vi "Warn.vi"(8 "Error In":errorcluster, 11 "Text":string) -> (0 "Error Out":errorcluster)   [LabVIEW 2014, in "Logger.lvlib"]
uses:
  Logger.lvlib
  Private/_Logger Action.ctl
  Controls/Message.ctl
  Controls/Tag.ctl
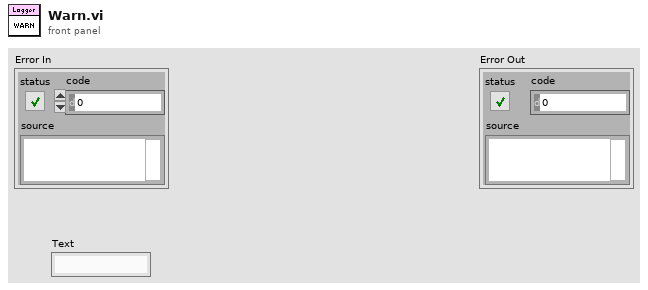
[diagram p1: front panel]
types:
  T1 = typedef "Logger.lvlib/Tag.ctl" = enum16{"Fatal", "Error", "Warn", "Info", "Debug", "Trace"}
  T2 = typedef "Logger.lvlib/_Logger Action.ctl" = enum16{"Initialize", "Register", "Log", "Unregister", "Set Level", "Shutdown"}
  T3 = typedef "Logger.lvlib/Message.ctl" = cluster{"Time Stamp":timestamp, "Tag":T1, "Source":string, "Text":string}
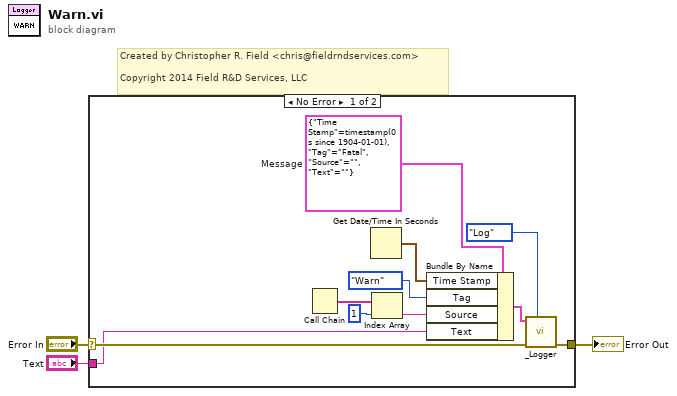
[diagram p0: block diagram]
diagram:
  # "Created by Christopher R. Field <chris@fieldrndservices.com>\n\nCopyright 2014 Field R&D Services, LLC"
  n1 = case shown="No Error" "Error In" {
    selector: "Error In" -> [w5 w15]
    tunnel: [w6 w15] -> w2
    tunnel: "Text" -> [w4 _]
    frame No Error {
      w11 = T3 {"Time Stamp"=timestamp(0 s since 1904-01-01), "Tag"=enum."Fatal", "Source"="", "Text"=""}  # Message
      n2 = Call Chain() -> (call chain=w13:string[])
      n3 = Get Date/Time In Seconds() -> (seconds since 1Jan1904=w10:timestamp)
      n4 = Index Array(array=w13, index=1) -> (element=w8:string)
      n5 = Bundle By Name(cluster=w11, "Time Stamp"=w10, "Tag"=Tag."Warn" ("Level"), "Source"=w8, "Text"=w4) -> (w7:T3)
      n6 = call "_Logger.vi"("Action"=_Logger_Action."Log", "Error In"=w5, "Value In"=w7) -> ("Error Out"=w6:errorcluster)  [unwired: 8 in]
    }
    frame Error {
    }
  }
  "Error Out" <- w2
